vi "Add Header Bytes.vi"(2 "Bytes/Msg":u64) -> (4 "Bytes/Msg with header":u64)   [LabVIEW 2021, in "ChannelCommon.lvlib"]
uses:
  ChannelCommon.lvlib
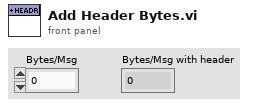
[diagram p1: front panel]
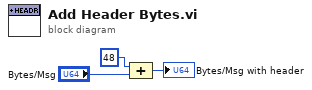
[diagram p0: block diagram]
diagram:
  n1 = Compound Arithmetic op=ADD(u64 48 ("value"), "Bytes/Msg") -> (→"Bytes/Msg with header":u64)
